vi "PPS Delimited string to numeric array.vi"(10 "delimiter":string="\t", 11 "1D string of numerics separated by delimiter":string="1\t2\t3\t4\t") -> (3 "Float array":dbl[](array[numeric])=[1.0, 2.0, 3.0, 4.0])   [LabVIEW 2016]
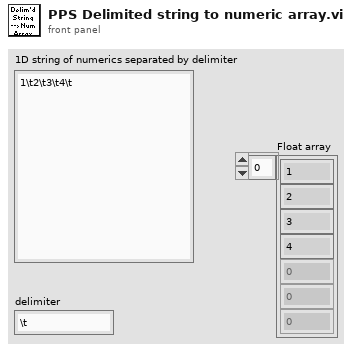
[diagram p1: front panel]
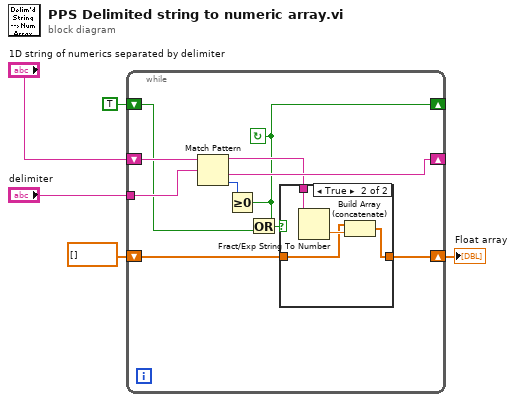
[diagram p0: block diagram]
diagram:
  n1 = while {
    shift-right: [w14] -> _
    shift-left: "1D string of numerics separated by delimiter" -> [w15]
    shift-right: [w10] -> w3
    shift-left: dbl[] [] -> [w11]
    tunnel: "delimiter" -> [w9]
    shift-right: [w8] -> _
    shift-left: TRUE -> [w7]
    stop <- w8 continue-if-true
    n2 = Match Pattern(string=w15, regular expression=w9) -> (before substring=w13:string, after substring=w14:string, offset past match=w12:i32)  [unwired: 1 in, 1 out]
    n3 = Greater Or Equal To 0?(x=w12) -> (x >= 0?=w8:bool)
    n4 = Or(x=w8, y=w7) -> (x .or. y?=w6:bool)
    n5 = case shown="True" w6 {
      tunnel: w13 -> [_ w20]
      tunnel: w11 -> [w16 w18]
      tunnel: [w16 w17] -> w10
      frame False {
      }
      frame True {
        n6 = Fract/Exp String To Number(string=w20) -> (number=w19:dbl)  [unwired: 3 in, 1 out]
        n7 = Build Array (concatenate)(w18, w19) -> (w17:dbl[])
      }
    }
  }
  "Float array" <- w3
